vi "BuildTable(SubVI).vi"(10 "String":string, 11 "UNDT_NTick":i32) -> (3 "Array":string[][](array[string]))   [LabVIEW 2017]
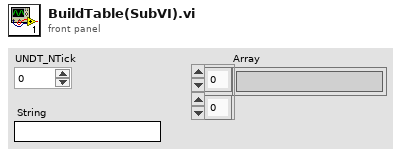
[diagram p1: front panel]
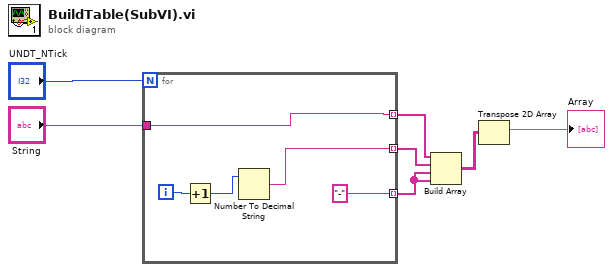
[diagram p0: block diagram]
diagram:
  n1 = for {
    N: "UNDT_NTick" -> [_]
    tunnel: [w11] -> w2 mode=indexing
    tunnel: ["-"] -> w5 mode=indexing
    tunnel: [w8] -> w4 mode=indexing
    tunnel: "String" -> [w8]
    i -> [w10]
    n2 = Increment(x=w10) -> (x+1=w9:i32)
    n3 = Number To Decimal String(number=w9) -> (decimal integer string=w11:string)  [unwired: 1 in]
  }
  n4 = Build Array(w4, w2, w5, w5) -> (w3:string[][])
  n5 = Transpose 2D Array(2D array=w3) -> (transposed array=→"Array":string[][])
